vi "Load Module.vi"(8 "error in":errorcluster, 10 "DB-Engine":refnum<class "DB-Interface.lvclass">, 11 "Config Section":string) -> (0 "error out":errorcluster, 3 "Module ID (dup)":i32)   [LabVIEW 2020, in "hse-db.lvlib" / "DB_CONNECTOR.lvlib"]
doc: "____\nHAMPEL SOFTWARE ENGINEERING v1.4.0 (2023-12-19 09:52)"
uses:
  DB_CONNECTOR.lvlib
  DB-Interface/DB-Interface.lvclass
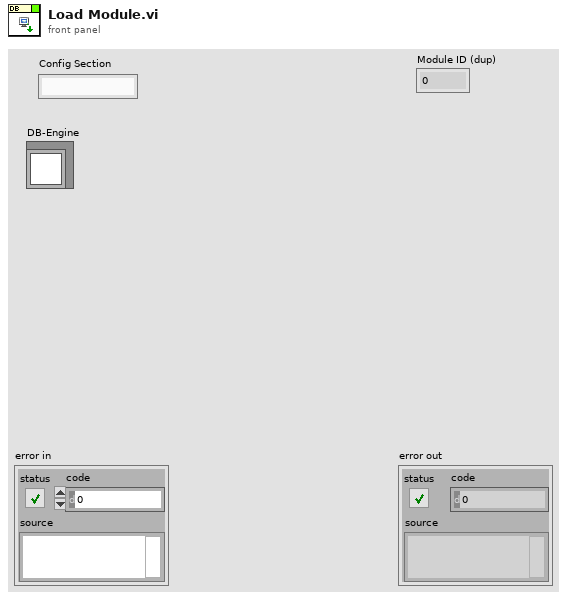
[diagram p1: front panel]
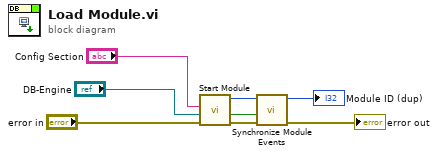
[diagram p0: block diagram]
diagram:
  n1 = call "Start Module.vi"("error in (no error)"="error in", "DB-Engine"="DB-Engine", "Config Section"="Config Section") -> ("error out"=w7:errorcluster, "Wait for Event Sync?"=w8:bool, "Module ID"=w6:i32)  [unwired: 5 in, 1 out]
  n2 = call "Synchronize Module Events.vi"("error in (no error)"=w7, "Wait for Event Sync?"=w8, "Module ID"=w6) -> ("error out"=→"error out":errorcluster, "Module ID (dup)"=→"Module ID (dup)":i32)  [unwired: 7 in]
